vi "PostScanAction.vi"(0 "Device en entrée":refnum<class "OR77200.lvclass"> caption="DNL_LabVIEW Object in", 5 "AcqComp":bool, 7 "ScanDev":bool caption="AcqComp", 11 "error in (no error)":errorcluster caption="entrée d'erreur (pas d'erreur)") -> (4 "Device en sortie":refnum<class "OR77200.lvclass"> caption="DNL_LabVIEW Object out", 6 "PostScanString":string, 15 "error out":errorcluster caption="sortie d'erreur")   [LabVIEW 2019, in "OR77200.lvclass"]
uses:
  OR77200.lvclass
  C:/Programmes Labview/LabscanV1A/DevicesClass/BaseDevice/BaseDevice.lvclass
  OR77200.lvclass/OR77200.ctl
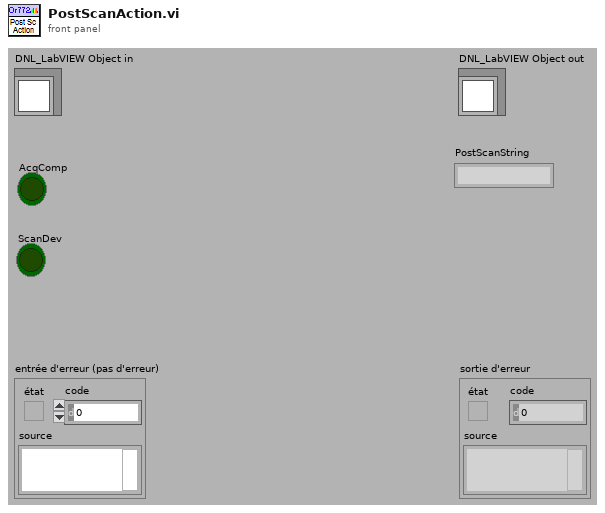
[diagram p1: front panel]
types:
  T1 = typedef "OR77200.lvclass/OR77200_Func.ctl" = enum16{"Position (nm)"}
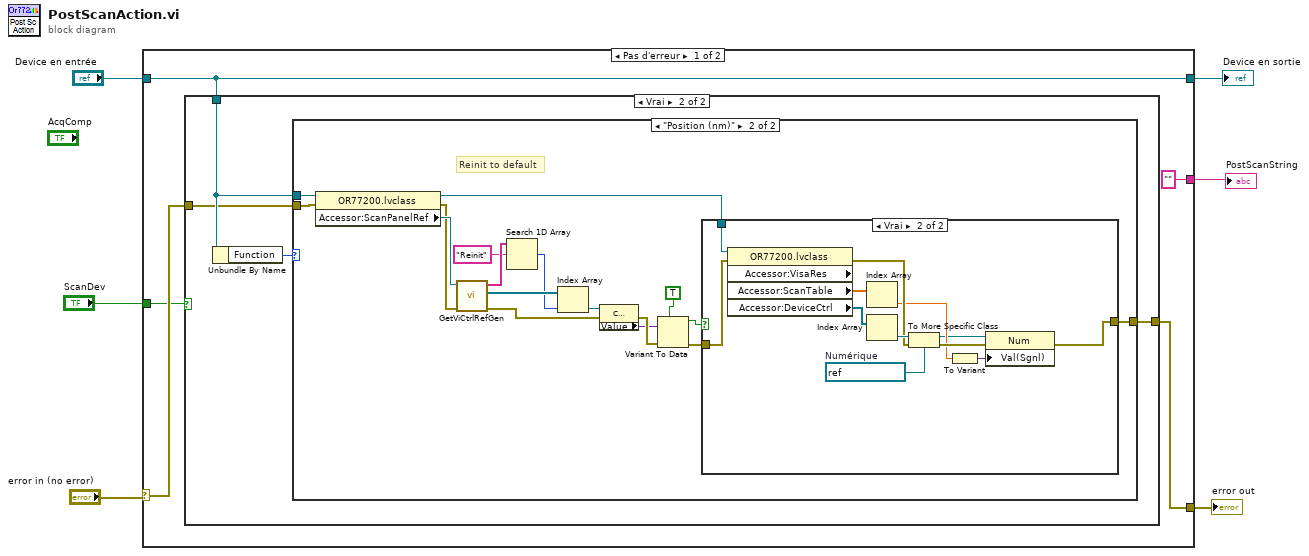
[diagram p0: block diagram]
diagram:
  n1 = case shown="Pas d'erreur" "error in (no error)" {
    selector: "error in (no error)" -> [w10 w48]
    tunnel: [w11 w49] -> w5
    tunnel: "Device en entrée" -> [w11 w49]
    tunnel: [w9 w48] -> w3
    tunnel: ["" _] -> w2
    tunnel: "ScanDev" -> [w7 _]
    frame No Error {
      n2 = case shown="Vrai" w7 {
        tunnel: w11 -> [_ w15]
        tunnel: w10 -> [w12 w14]
        tunnel: [w12 w13] -> w9
        frame False {
        }
        frame True {
          n3 = Unbundle By Name(w15) -> ("Function"=w16:T1)
          n4 = case shown="\"Position (nm)\"" w16 {
            tunnel: w15 -> [_ w34]
            tunnel: w14 -> [w17 w33]
            tunnel: [w17 w18] -> w13
            frame Default {
            }
            frame "Position (nm)" {
              # "Reinit to default"
              n5 = property class="OR77200.lvclass"(reference=w34, error in=w33) -> (reference out=w20:refnum<class "OR77200.lvclass">, error out=w28:errorcluster, "Accessor:ScanPanelRef"=w32:refnum<vi>)
              n6 = call <userlib>:"GetViCtrlRefGen.vi"("ErrorIn(No Error)"=w28, "VIRef"=w32) -> ("sortie d'erreur"=w29:errorcluster, "ControlsRefs"=w31:refnum<vi>[], "ControlsNames"=w24:string[])  [unwired: 7 in]
              n7 = Search 1D Array(1D array=w24, element="Reinit" ("élément")) -> (index of element=w22:i32)  [unwired: 1 in]
              n8 = Index Array(array=w31, index=w22) -> (element=w30:refnum<vi>)
              n9 = property class="Cmde"(reference=w30, error in=w29) -> (error out=w27:errorcluster, "Value"=w26:variant)  [unwired: 1 out]
              n10 = Variant To Data(error in=w27, type=TRUE ("Valeur"), Variant=w26) -> (data=w21:bool, error out=w19:errorcluster)
              n11 = case shown="Vrai" w21 {
                tunnel: w20 -> [_ w47]
                tunnel: w19 -> [w35 w45]
                tunnel: [w35 w37] -> w18
                frame False {
                }
                frame True {
                  w43 = refnum<vi> refnum  # Numérique
                  n12 = property class="OR77200.lvclass" props=["Accessor:VisaRes", "Accessor:ScanTable", "Accessor:DeviceCtrl"](reference=w47, error in=w45) -> (error out=w41:errorcluster, "Accessor:ScanTable"=w46:dbl[], "Accessor:DeviceCtrl"=w42:refnum<vi>[])  [unwired: 2 out]
                  n13 = Index Array(array=w46) -> (element=w39:dbl)  [unwired: 1 in]
                  n14 = Index Array(array=w42) -> (element=w44:refnum<vi>)  [unwired: 1 in]
                  n15 = To More Specific Class(target class=w43, reference=w44, error in=w41) -> (specific class reference=w36:refnum<vi>, error out=w40:errorcluster)
                  n16 = To Variant(anything=w39) -> (Variant=w38:variant)
                  n17 = property class="Num"(reference=w36, error in=w40, "Val(Sgnl)"=w38) -> (error out=w37:errorcluster)  [unwired: 1 out]
                }
              }
            }
          }
        }
      }
    }
    frame Error {
    }
  }
  "error out" <- w3
  "Device en sortie" <- w5
  "PostScanString" <- w2
